vi "Extract Output Terminals.vi"(8 "error in (no error)":errorcluster, 11 "Array in":refnum<vi>[](array[refnum])) -> (0 "error out":errorcluster, 1 "parameters":string, 2 "defaults string":string, 3 "names string":string)   [LabVIEW 2025, in "Scripting Server.lvlib"]
uses:
  Scripting Server.lvlib
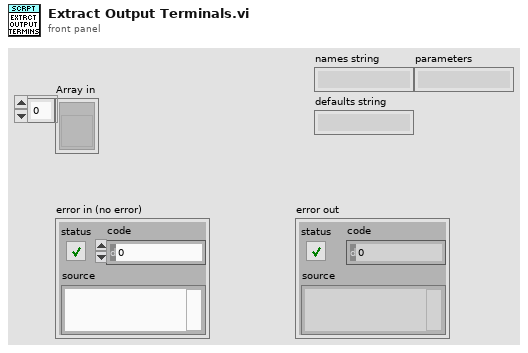
[diagram p1: front panel]
types:
  T1 = typedef "Datatypes.ctl" = enum16{"Float", "Int", "String", "Bool", "Invalid"}
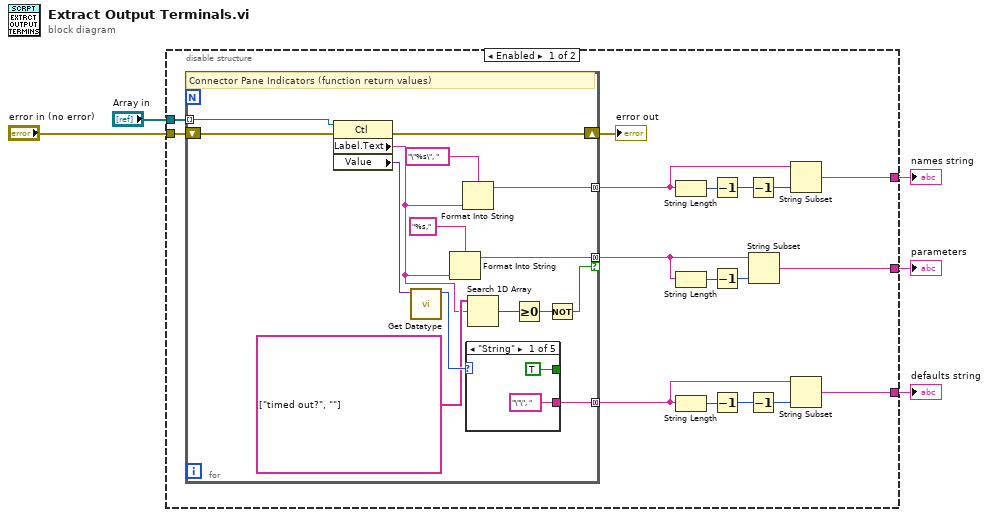
[diagram p0: block diagram]
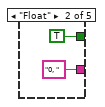
[diagram p2: hidden frame]
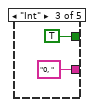
[diagram p3: hidden frame]
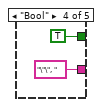
[diagram p4: hidden frame]
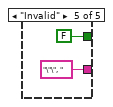
[diagram p5: hidden frame]
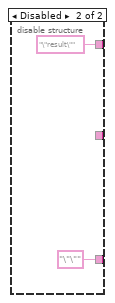
[diagram p6: hidden frame]
diagram:
  n1 = disable-structure shown="Enabled" {
    disable-tunnel: "error in (no error)" -> [w22 _]
    disable-tunnel: "Array in" -> [w21 _]
    disable-tunnel: [w16 "\"result\"" ("names string")] -> w3
    disable-tunnel: [w12 "\"\"" ("defaults string")] -> w2
    disable-tunnel: [w7 _] -> w1
    frame Enabled {
      n2 = for {
        tunnel: w21 -> [w35] mode=indexing
        shift-right: [w36] -> w20
        shift-left: w22 -> [w37]
        tunnel: [w33] -> w17 mode=concatenating
        tunnel: [w30] -> w13 mode=concatenating
        tunnel: [w25] -> w10 mode=concatenating if=w23
        # "Connector Pane Indicators (function return values)"
        n3 = property class="Ctl"(reference=w35, error in=w37) -> (error out=w36:errorcluster, "Label.Text"=w26:string, "Value"=w32:variant)  [unwired: 1 out]
        n4 = call "Get Datatype.vi"("Value"=w32) -> ("datatypes"=w31:T1)  [unwired: 10 in]
        n5 = Format Into String(format string="%s,", w26) -> (resulting string=w25:string)  [unwired: 2 in, 1 out]
        n6 = Format Into String(format string="\"%s\", ", w26) -> (resulting string=w33:string)  [unwired: 2 in, 1 out]
        n7 = case shown="\"String\"" w31 {
          tunnel: [TRUE TRUE TRUE TRUE FALSE] -> _
          tunnel: ["\"\", " ("format string") "0, " ("format string") "0, " ("format string") "\"\", " ("format string") "\"\", " ("format string")] -> w30
          frame "String" {
          }
          frame "Float" {
          }
          frame "Int" {
          }
          frame "Bool" {
          }
          frame "Invalid" {
          }
        }
        n8 = Search 1D Array(1D array=string[] ["timed out?", ""], element=w26) -> (index of element=w29:i32)  [unwired: 1 in]
        n9 = Greater Or Equal To 0?(x=w29) -> (x >= 0?=w24:bool)
        n10 = Not(x=w24) -> (.not. x?=w23:bool)
      }
      "error out" <- w20
      n11 = String Length(string=w17) -> (length=w18:i32)
      n12 = String Length(string=w10) -> (length=w9:i32)
      n13 = String Length(string=w13) -> (length=w15:i32)
      n14 = Decrement(x=w18) -> (x-1=w6:i32)
      n15 = Decrement(x=w9) -> (x-1=w8:i32)
      n16 = Decrement(x=w15) -> (x-1=w14:i32)
      n17 = Decrement(x=w6) -> (x-1=w19:i32)
      n18 = Decrement(x=w14) -> (x-1=w11:i32)
      n19 = String Subset(string=w10, length (rest)=w8) -> (substring=w7:string)  [unwired: 1 in]
      n20 = String Subset(string=w17, length (rest)=w19) -> (substring=w16:string)  [unwired: 1 in]
      n21 = String Subset(string=w13, length (rest)=w11) -> (substring=w12:string)  [unwired: 1 in]
    }
    frame Disabled {
    }
  }
  "names string" <- w3
  "defaults string" <- w2
  "parameters" <- w1
